vi "Get Latest Message Tracker.vi"(8 "error in (no error)":errorcluster, 11 "Debugger in":refnum<class "Debugger.lvclass">) -> (0 "error out":errorcluster, 2 "Log":refnum<class "Debug Log.lvclass">, 3 "Debugger out":refnum<class "Debugger.lvclass">)   [LabVIEW 2020, in "Debugger.lvclass"]
uses:
  Debugger.lvclass
  Debug Log/Debug Log.lvclass
  Debugger.lvclass/Debugger.ctl
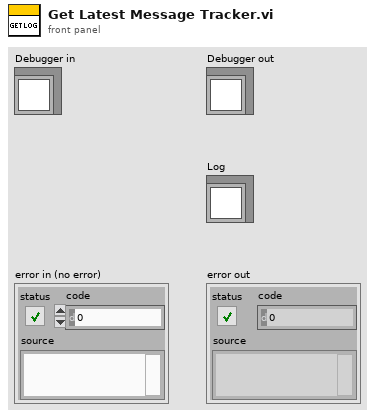
[diagram p1: front panel]
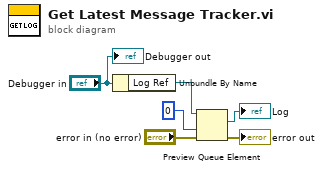
[diagram p0: block diagram]
diagram:
  n1 = Unbundle By Name("Debugger in") -> ("Log Ref"=w5:refnum<queue>)
  n2 = Preview Queue Element(queue=w5, timeout in ms (-1)=0, error in (no error)="error in (no error)") -> (element=→"Log":refnum<class "Debug Log.lvclass">, error out=→"error out":errorcluster)  [unwired: 2 out]
  "Debugger out" <- "Debugger in"
